vi "LS372_read_only_Quwue_Commands.vi"(1 "LS372_only_read-Cluster Control":T1, 3 "Queue":refnum<queue>) -> (0 "LS372_only_read-Cluster Control new Status":T1)   [LabVIEW 2019]
uses:
  LS372/LS372_read_only-Control.ctl
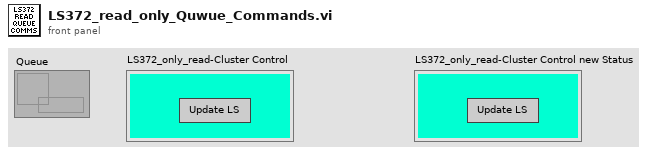
[diagram p1: front panel]
types:
  T1 = typedef "LS372_read_only-Control.ctl" = cluster{"Update Lakeshores":bool}
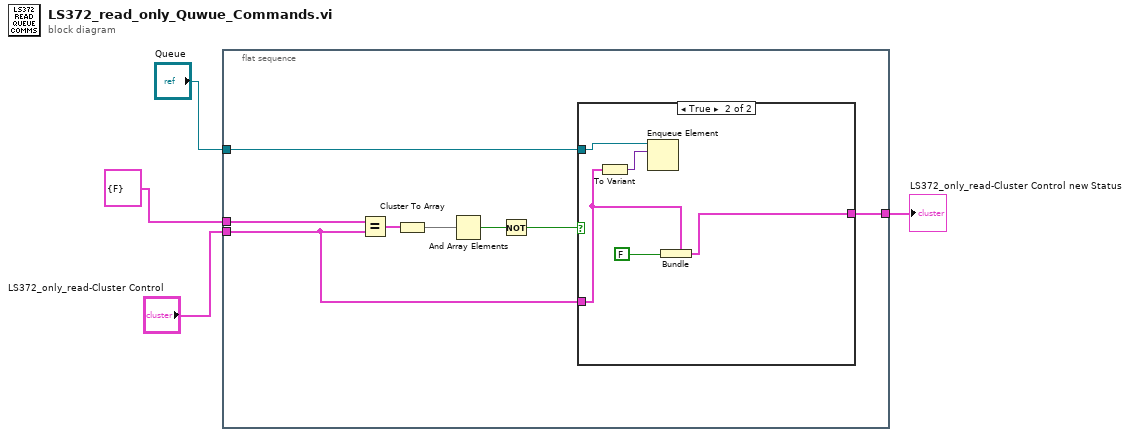
[diagram p0: block diagram]
diagram:
  n1 = flat-sequence {
    tunnel: T1 {"Update Lakeshores"=FALSE} ("LS372_only_read-Cluster Control") -> [w12]
    tunnel: "LS372_only_read-Cluster Control" -> [w7]
    tunnel: "Queue" -> [w6]
    tunnel: [w5] -> w1
    frame #0 {
      n2 = Equal?(x=w12, y=w7) -> (x = y?=w11:T1)
      n3 = Cluster To Array(cluster=w11) -> (array=w10:bool[])
      n4 = And Array Elements(Boolean array=w10) -> (logical AND=w9:bool)
      n5 = Not(x=w9) -> (.not. x?=w8:bool)
      n6 = case shown="True" w8 {
        tunnel: w7 -> [w13 w16]
        tunnel: w6 -> [_ w18]
        tunnel: [w13 w14] -> w5
        frame False {
        }
        frame True {
          n7 = To Variant(anything=w16) -> (Variant=w17:variant)
          n8 = Enqueue Element(queue=w18, element=w17) -> ()  [unwired: 2 in, 3 out]
          n9 = Bundle(cluster=w16, "Update Lakeshores"=FALSE) -> (w14:T1)
        }
      }
    }
  }
  "LS372_only_read-Cluster Control new Status" <- w1
